vi "traffic light  temperatre indication.vi"() -> ()   [LabVIEW 2018]
panel:
  in  "current temp 2":u8
  in  "reset 2":bool
  out "max temp  2":u8
  in  "stop 3":bool
  out "clock cycle  2":i32
  out "min temp   2":u8
  in  "stop":bool
  in  "yellow time  2":dbl
  in  "green time":dbl
  in  "yellow time":dbl
  in  "red time":dbl
  out "time":dbl
  out "green":bool
  out "yellow":bool
  out "red":bool
  # "the  first  part  in  the  project  traffic  light"
  # "the second part in the project temperature indicator"
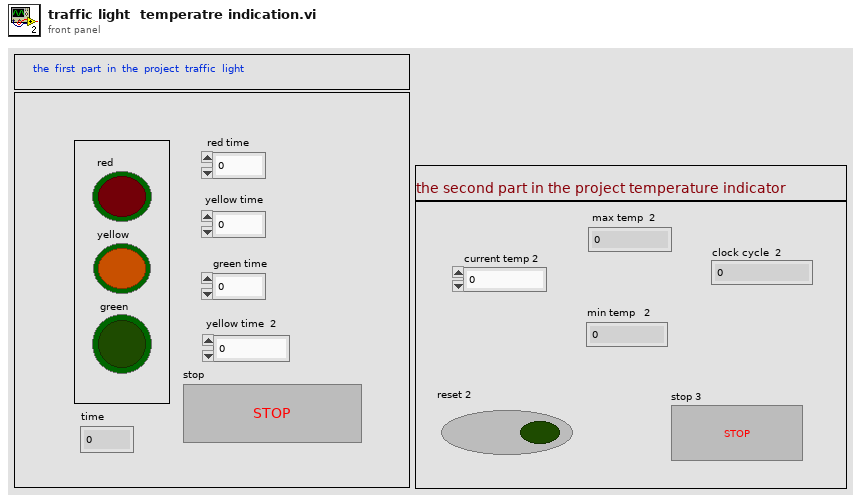
[diagram p1: front panel]
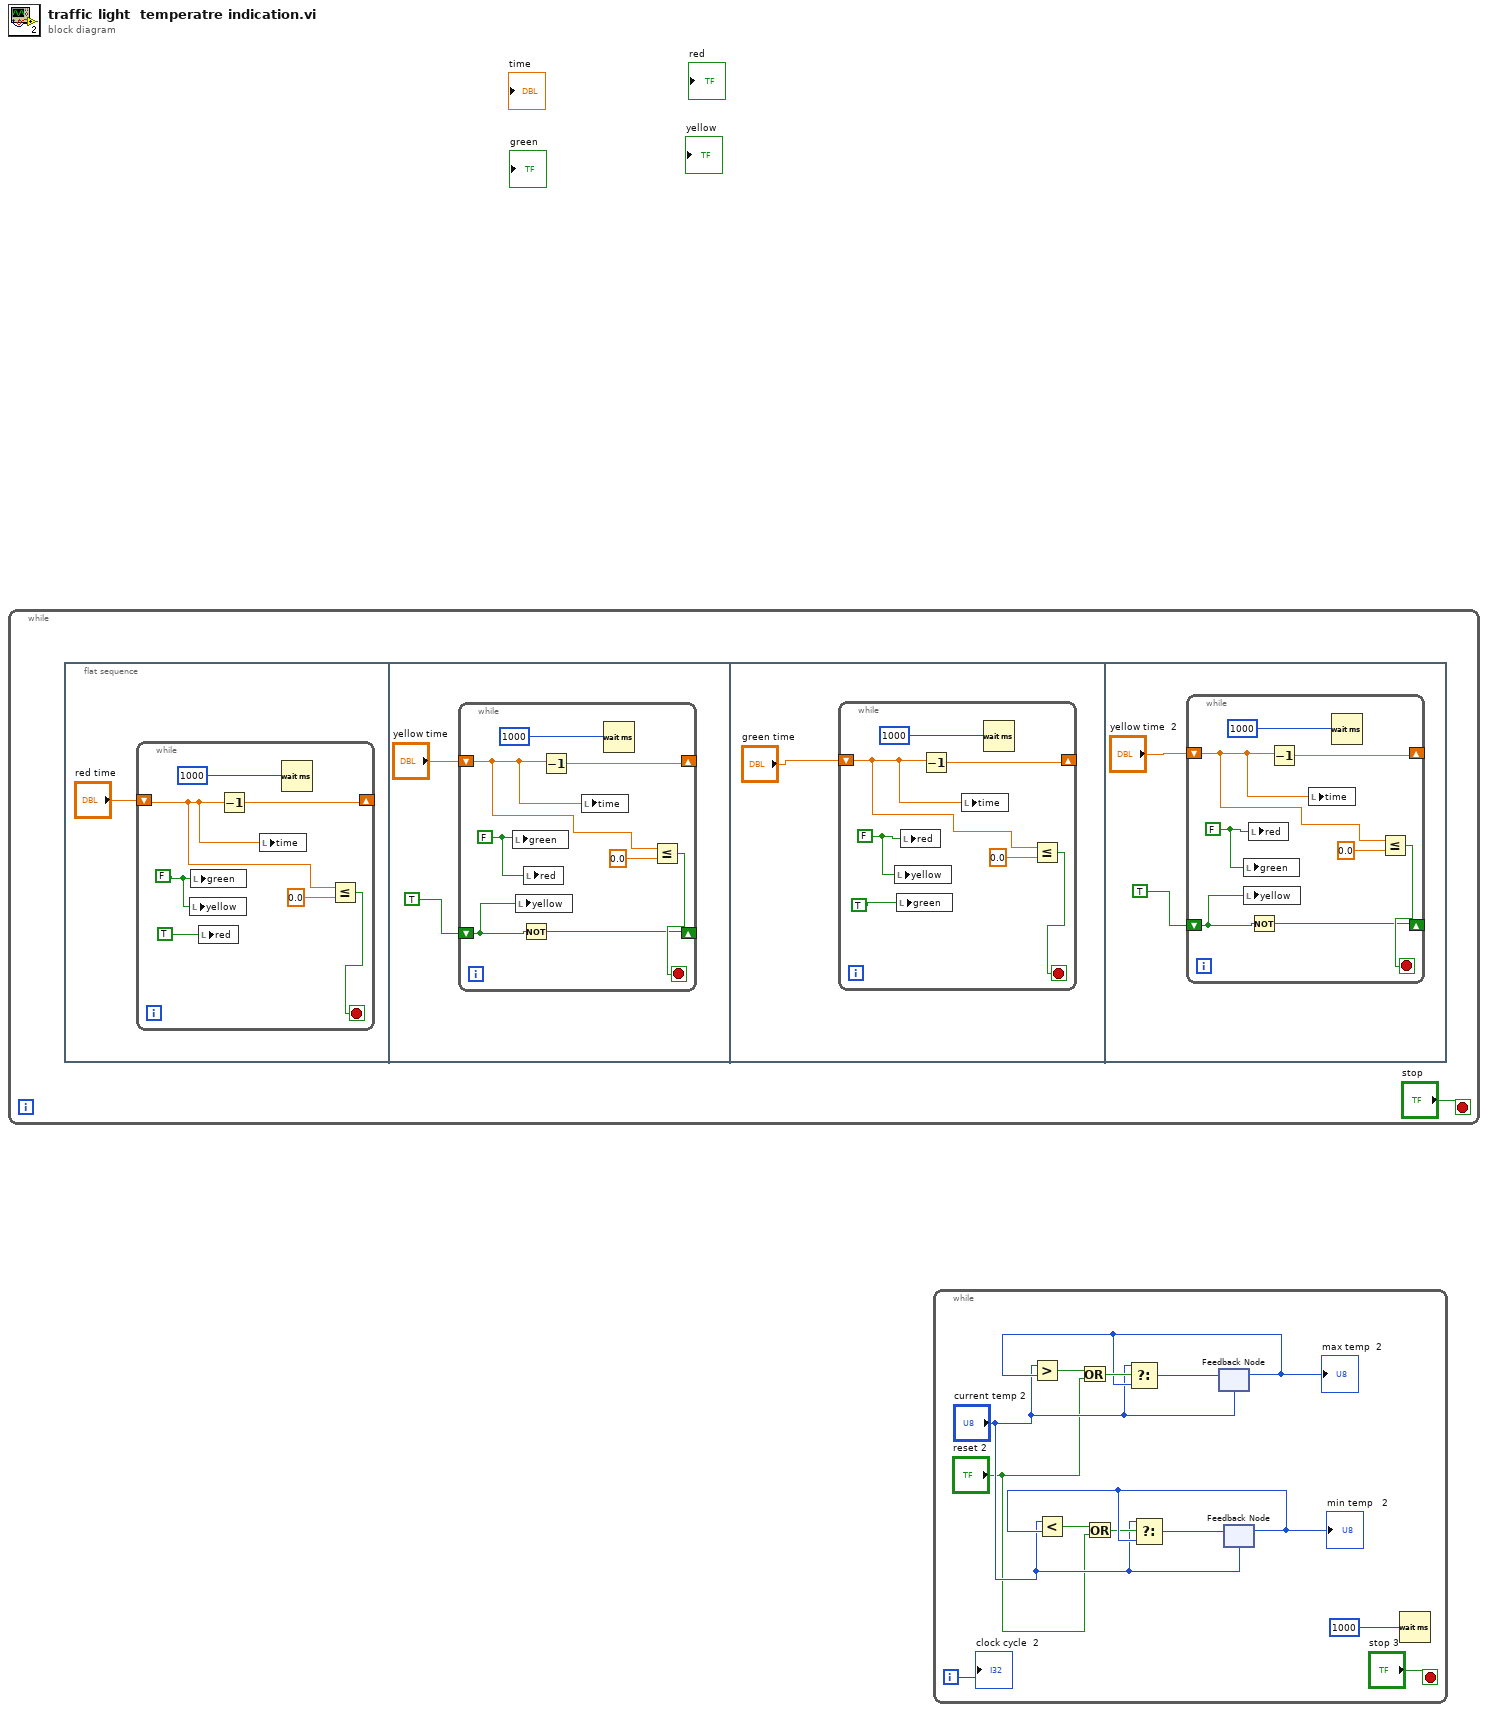
[diagram p0: block diagram]
diagram:
  n1 = while {
    stop <- "stop" stop-if-true
    n2 = flat-sequence {
      frame #0 {
        n3 = while {
          shift-right: [w7] -> _
          shift-left: "red time" -> [w6]
          stop <- w4 stop-if-true
          w9 = FALSE
          n4 = local write "yellow"(w9) -> ()
          n5 = local write "green"(w9) -> ()
          n6 = local write "red"(TRUE ("red")) -> ()
          n7 = Decrement(x=w6) -> (x-1=w7:dbl)
          n8 = local write "time"(w6) -> ()
          n9 = Wait (ms)(milliseconds to wait=u32 1000 ("millisecond timer value")) -> ()  [unwired: 1 out]
          n10 = Less Or Equal?(x=w6, y=0.0) -> (x <= y?=w4:bool)
        }
      }
      frame #1 {
        n11 = while {
          shift-right: [w19] -> _
          shift-left: "yellow time" -> [w12]
          shift-right: [w14] -> _
          shift-left: TRUE ("red") -> [w13]
          stop <- w17 stop-if-true
          w15 = FALSE
          n12 = local write "green"(w15) -> ()
          n13 = local write "yellow"(w13) -> ()
          n14 = Not(x=w13) -> (.not. x?=w14:bool)
          n15 = local write "red"(w15) -> ()
          n16 = Decrement(x=w12) -> (x-1=w19:dbl)
          n17 = local write "time"(w12) -> ()
          n18 = Wait (ms)(milliseconds to wait=u32 1000 ("millisecond timer value")) -> ()  [unwired: 1 out]
          n19 = Less Or Equal?(x=w12, y=0.0) -> (x <= y?=w17:bool)
        }
      }
      frame #2 {
        n20 = while {
          shift-right: [w27] -> _
          shift-left: "green time" -> [w22]
          stop <- w25 stop-if-true
          w23 = FALSE
          n21 = local write "yellow"(w23) -> ()
          n22 = local write "green"(TRUE ("red")) -> ()
          n23 = local write "red"(w23) -> ()
          n24 = Decrement(x=w22) -> (x-1=w27:dbl)
          n25 = local write "time"(w22) -> ()
          n26 = Wait (ms)(milliseconds to wait=u32 1000 ("millisecond timer value")) -> ()  [unwired: 1 out]
          n27 = Less Or Equal?(x=w22, y=0.0) -> (x <= y?=w25:bool)
        }
      }
      frame #3 {
        n28 = while {
          shift-right: [w37] -> _
          shift-left: "yellow time  2" -> [w30]
          shift-right: [w32] -> _
          shift-left: TRUE ("red") -> [w31]
          stop <- w35 stop-if-true
          w33 = FALSE
          n29 = local write "green"(w33) -> ()
          n30 = local write "yellow"(w31) -> ()
          n31 = local write "red"(w33) -> ()
          n32 = Not(x=w31) -> (.not. x?=w32:bool)
          n33 = Decrement(x=w30) -> (x-1=w37:dbl)
          n34 = local write "time"(w30) -> ()
          n35 = Wait (ms)(milliseconds to wait=u32 1000 ("millisecond timer value")) -> ()  [unwired: 1 out]
          n36 = Less Or Equal?(x=w30, y=0.0) -> (x <= y?=w35:bool)
        }
      }
    }
  }
  n37 = while {
    i -> [w45]
    stop <- "stop 3" stop-if-true
    n38 = feedback #1("current temp 2") -> (w48:u8)
    "max temp  2" <- w48
    n39 = Greater?(x="current temp 2", y=w48) -> (0:w49:bool)
    n40 = Or(x=w49, y="reset 2") -> (x .or. y?=w50:bool)
    n41 = Select(t="current temp 2", s=w50, f=w48) -> (s? t:f=w47:u8)
    n42 = feedback-in #1(w47) -> ()
    n43 = feedback #2("current temp 2") -> (w42:u8)
    "min temp   2" <- w42
    n44 = Less?(x="current temp 2", y=w42) -> (x < y?=w41:bool)
    n45 = Or(x=w41, y="reset 2") -> (x .or. y?=w40:bool)
    n46 = Select(t="current temp 2", s=w40, f=w42) -> (s? t:f=w43:u8)
    n47 = feedback-in #2(w43) -> ()
    n48 = Wait (ms)(milliseconds to wait=u32 1000) -> ()  [unwired: 1 out]
    "clock cycle  2" <- w45
  }
